vi "Post Substeps Analog Output Task.vi"(9 "AOWrite":T1, 10 "Socket No":u16=1, 11 "Sequence Context In":refnum<k7>) -> (0 "error out":errorcluster, 2 "PhysicalChannel":string[](array[string]), 3 "Report Text":string)   [LabVIEW 2023, in "LTT_TeststandSteptypes.lvlib"]
doc: "This VI Is Socket Number based AO Data Signal Write Through Q"
uses:
  LTT_TeststandSteptypes.lvlib
  HardwareAbstractionLayer_LVOOP/Main/Class Options.ctl
  HardwareAbstractionLayer_LVOOP/Analog Output/AO/AO.lvclass
  HardwareAbstractionLayer_LVOOP/Main/Main.lvclass
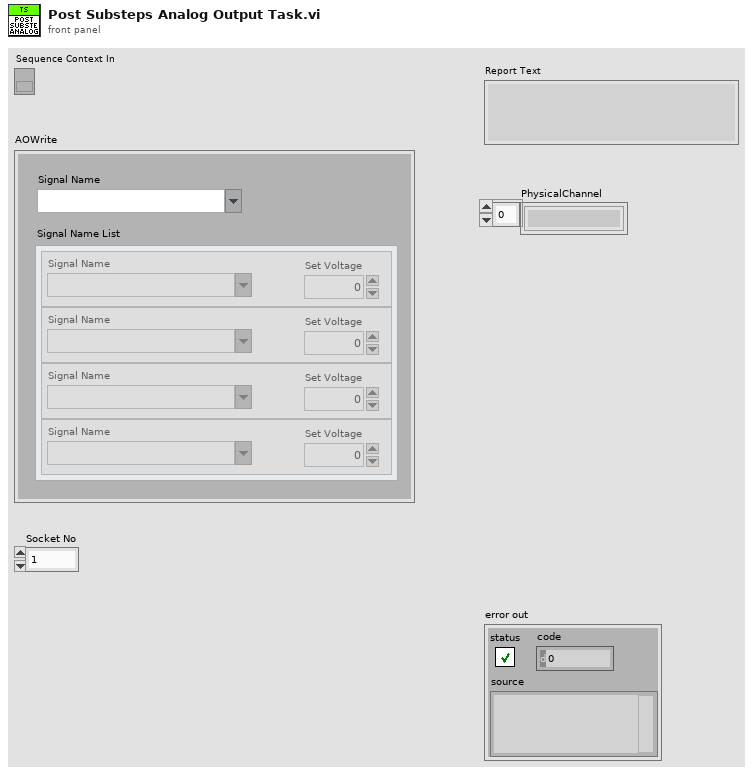
[diagram p1: front panel]
types:
  T1 = cluster{"Signal Name":string, "Signal Name List":cluster{"Signal Name":string, "Set Voltage":dbl}[]}
  T2 = typedef "HardwareAbstractionLayer_LVOOP.lvlib/Main.lvclass/Class Options.ctl" = enum16{"Init All Class", "Read All Class", "Write AI Class", "Write AO Class", "Write AO Waveform Generation", "Write DI Class", "Write DO Class", "Write PWM Input Class", "Write PWM Output Class", "Exit"}
  T3 = typedef "HardwareAbstractionLayer_LVOOP.lvlib/Main.lvclass/Class Ref.ctl" = cluster{"FGV":refnum<class "Function Global Variable.lvclass">, "Notifier":refnum<class "NotifierHandler.lvclass">, "Queue":refnum<class "Queue Handler.lvclass">, "User Event":refnum<class "User Event.lvclass">, "Data Manager":refnum<class "Data Manager.lvclass">, "DMM":refnum<class "DMM.lvclass">, "Function Generator":refnum<class "Function Generator.lvclass">, "Oscilloscope":refnum<class "Oscilloscope.lvclass">, "PowerSupply":refnum<class "PowerSupply.lvclass">, "Teststand":refnum<class "Teststand.lvclass">, "AO":refnum<class "AO.lvclass">, "AI":refnum<class "AI.lvclass">, "Database":refnum<class "Database.lvclass">, "AO Waveform Generation":refnum<class "AO.lvclass">, "DO":refnum<class "DO.lvclass">, "DI":refnum<class "DI.lvclass">, "PWM Output":refnum<class "PWM Output.lvclass">, "PWM Input":refnum<class "PWM Input.lvclass">, "RelayOutput":refnum<class "NISwitch.lvclass">, "Modbus":refnum<class "Modbus.lvclass">, "CAN":refnum<class "CAN.lvclass">}
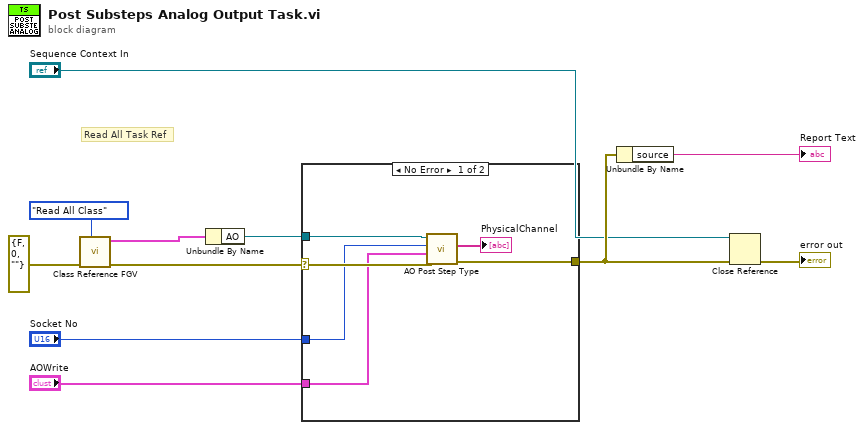
[diagram p0: block diagram]
diagram:
  # "Read All Task Ref"
  n1 = call "Class Reference FGV.vi"("Options"=Class_Options."Read All Class", "error in"=errorcluster {"status"=FALSE, "code"=0, "source"=""}) -> ("error out"=w4:errorcluster, "Class Cluster Out"=w2:T3)  [unwired: 8 in]
  n2 = Unbundle By Name(w2) -> ("AO"=w1:refnum<class "AO.lvclass">)
  n3 = case shown="No Error" w4 {
    selector: w4 -> [w16 w18]
    tunnel: [w15 w18] -> w10
    tunnel: "AOWrite" -> [w13 _]
    tunnel: "Socket No" -> [w14 _]
    tunnel: w1 -> [w17 _]
    frame No Error {
      n4 = call-dynamic "AO Post Step Type.vi"("error in (no error)"=w16, "AOWrite"=w13, "Socket No"=w14, "AO in"=w17) -> ("error out"=w15:errorcluster, "PhysicalChannel"=→"PhysicalChannel":string[])  [unwired: 5 in, 1 out]
    }
    frame Error {
    }
  }
  n5 = Unbundle By Name(w10) -> ("source"=→"Report Text":string)
  n6 = Close Reference(reference="Sequence Context In", error in (no error)=w10) -> (error out=→"error out":errorcluster)
